vi "Create.vi"(7 "mode settings":variant, 8 "error in":errorcluster, 9 "number of default channels":i32, 10 "channel settings":variant, 11 "counter input PWM mode in":refnum<class "Counter Input PWM Mode.lvclass">) -> (0 "error out":errorcluster, 1 "channels":refnum<class "Channel.lvclass">[](array[class]), 3 "counter input PWM mode out":refnum<class "Counter Input PWM Mode.lvclass">)   [LabVIEW 2020, in "Scan Engine Scripting.lvlib" / "Counter Input PWM Mode.lvclass"]
uses:
  Counter Input PWM Mode.lvclass
  Channel Classes/Channel/Channel.lvclass
  Controls/counter input pwm channel settings.ctl
  Channel Classes/PWM Input Channel/Measurement Type.ctl
  f5685796-a93e-4056-970a-a8238cbbc772.vi
  Channel Classes/PWM Input Channel/PWM Input Channel.lvclass
  C:/jenkins/workspace/ercat-custom-device_release_20.4/Custom Device Source/Scripting/Modules/Channel Classes/Channel/Channel.lvclass
  Scan Engine Scripting.lvlib
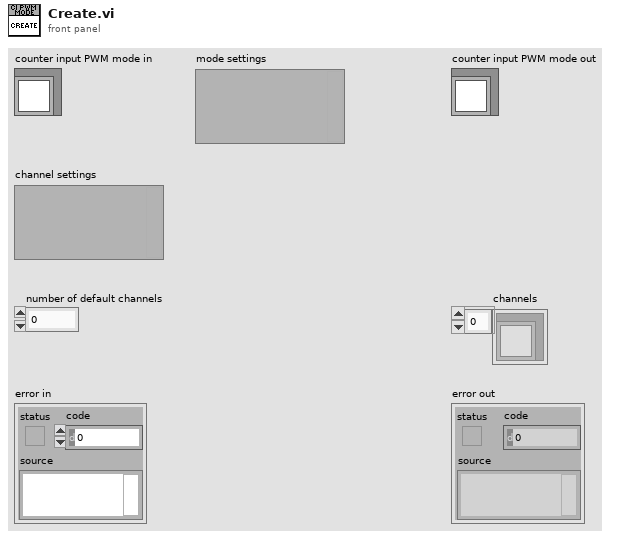
[diagram p1: front panel]
types:
  T1 = typedef "Scan Engine Scripting.lvlib/counter input pwm channel settings.ctl" = cluster{"name":string, "default value":dbl, "measurement type":T2}
  T2 = typedef "Scan Engine Scripting.lvlib/PWM Input Channel.lvclass/Measurement Type.ctl" = enum16{"High Pulse", "Low Pulse", "Most Recent"}
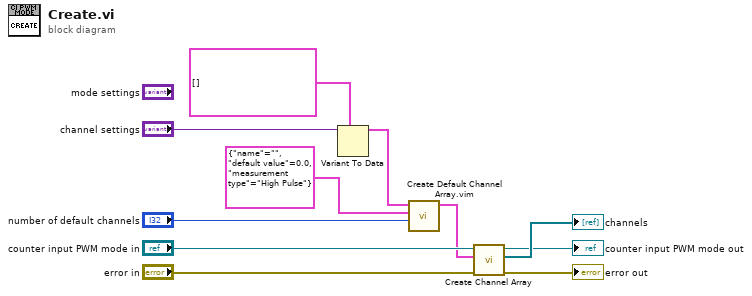
[diagram p0: block diagram]
diagram:
  n1 = Variant To Data(type=T1[] [], Variant="channel settings") -> (data=w9:T1[])  [unwired: 1 in, 1 out]
  n2 = call "Create Default Channel Array.vim"("number of default channels"="number of default channels", "default settings"=T1 {"name"="", "default value"=0.0, "measurement type"=enum."High Pulse"} ("channel settings"), "channel settings in"=w9) -> ("channel settings out"=w2:T1[])  [unwired: 8 in]
  n3 = call "Create Channel Array.vi"("error in"="error in", "channel settings"=w2, "counter input PWM mode in"="counter input PWM mode in") -> ("error out"=→"error out":errorcluster, "channels"=→"channels":refnum<class "PWM Input Channel.lvclass">[], "counter input PWM mode out"=→"counter input PWM mode out":refnum<class "Counter Input PWM Mode.lvclass">)  [unwired: 6 in]
